vi "Create.vi"(8 "error in (no error)":errorcluster, 10 "Cylinder Types":T1, 11 "Actuator Cylinder Factory in":refnum<class "Actuator Cylinder Factory.lvclass">) -> (0 "error out":errorcluster, 2 "Actuator Cylinder":refnum<class "Actuator Cylinder.lvclass">, 3 "Actuator Cylinder Factory out":refnum<class "Actuator Cylinder Factory.lvclass">)   [LabVIEW 2015, in "Actuator Cylinder Factory.lvclass"]
uses:
  Actuator Cylinder Factory.lvclass
  Actuator Cylinder/Actuator Cylinder.lvclass
  Typedefs/Cylinder Types.ctl
  ILC DAC/ILC DAC Factory/ILC DAC Factory.lvclass
  ILC PSV Open Loop Actuator Cylinder/ILC PSV Open Loop Actuator Cylinder.lvclass
  ILC PSV Closed Loop Actuator Cylinder/ILC PSV Closed Loop Actuator Cylinder.lvclass
  ILC TV Open Loop Actuator Cylinder/ILC TV Open Loop Actuator Cylinder.lvclass
  ILC TV Closed Loop Actuator Cylinder/ILC TV Closed Loop Actuator Cylinder.lvclass
  ILC Closed Loop Actuator Cylinder/ILC Closed Loop Actuator Cylinder.lvclass
  ILC Actuator Cylinder/ILC Actuator Cylinder.lvclass/ILC Actuator Cylinder.ctl
  ILC Actuator Cylinder/ILC Actuator Cylinder.lvclass
  Boot Loader/Boot Loader.lvclass
  Typedefs/FAMT Typedefs.lvlib
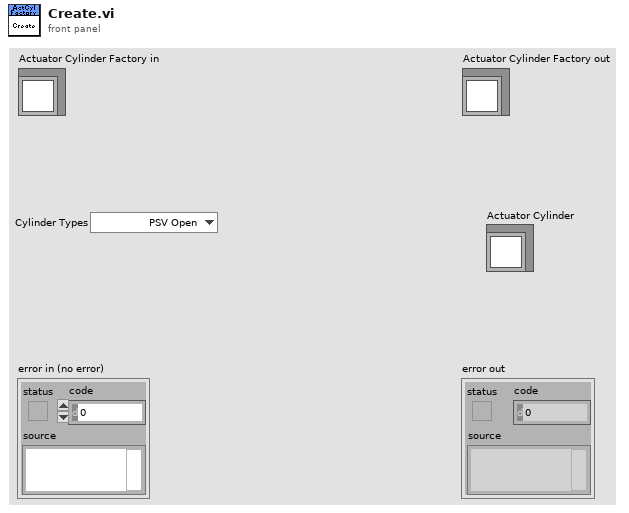
[diagram p1: front panel]
types:
  T1 = typedef "FAMT Typedefs.lvlib/Cylinder Types.ctl" = enum16{"PSV Open", "PSV Closed", "TV Open", "TV Closed", "Closed"}
  T2 = typedef "FAMT Typedefs.lvlib/Connection Settings.ctl" = cluster{"Pressure Servo Valve 1 DAC":u8, "Pressure Servo Valve 2 DAC":u8, "Flow Control Valve DAC":u8, "Load Cell ADC":u8, "FC1 ILC Port":refnum<visa-resource-name>, "FC2 ILC Port":refnum<visa-resource-name>, "Tovey A-B Port":refnum<visa-resource-name>, "Tovey C-D Port":refnum<visa-resource-name>, "Tovey E-F Port":refnum<visa-resource-name>, "FC1 ILC Protocol":T3, "FC2 ILC Protocol":T3, "Tovey A-B Protocol":T3, "Tovey C-D Protocol":T3, "Tovey E-F Protocol":T3, "Tovey A-B Address":u8, "Tovey C-D Address":u8, "Tovey E-F Address":u8}
  T3 = typedef "SerialProtocols.lvlib/SerialProtocol.ctl" = enum16{"RS232", "RS485", "SerialSimulator"}
  T4 = typedef "FAMT Typedefs.lvlib/Pressure Servo Valve Settings.ctl" = cluster{"Center Point":dbl[unit], "Area":dbl, "PA to PSI":dbl, "Off Value":dbl}
  T5 = typedef "FAMT Typedefs.lvlib/Turbo Valve Settings.ctl" = cluster{"ROT Bias":u8, "Minimum Voltage":dbl, "Maximum Voltage":dbl, "Off Value":dbl}
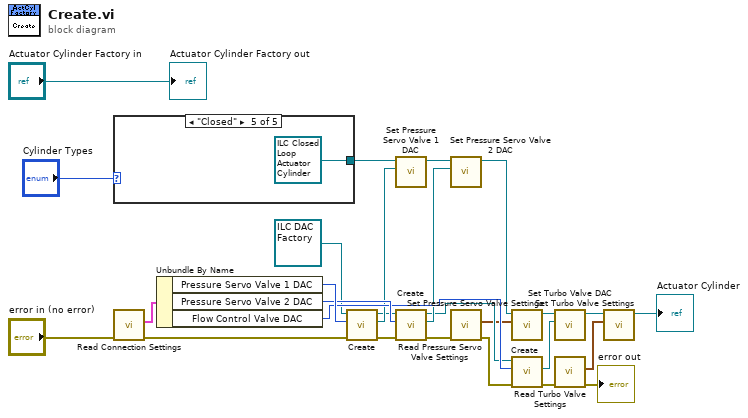
[diagram p0: block diagram]
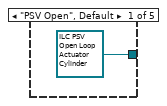
[diagram p2: hidden frame]
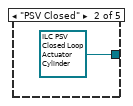
[diagram p3: hidden frame]
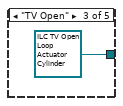
[diagram p4: hidden frame]
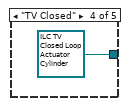
[diagram p5: hidden frame]
diagram:
  n1 = case shown="\"Closed\"" "Cylinder Types" {
    tunnel: [refnum<class "ILC PSV Open Loop Actuator Cylinder.lvclass"> refnum ("ILCPSVOpenLoopActuatorCylinder.lvclass") refnum<class "ILC PSV Closed Loop Actuator Cylinder.lvclass"> refnum ("ILCPSVClosedLoopActuatorCylinder.lvclass") refnum<class "ILC TV Open Loop Actuator Cylinder.lvclass"> refnum ("ILCTVOpenLoopActuatorCylinder.lvclass") refnum<class "ILC TV Closed Loop Actuator Cylinder.lvclass"> refnum ("ILCTVClosedLoopActuatorCylinder.lvclass") refnum<class "ILC Closed Loop Actuator Cylinder.lvclass"> refnum ("ILCClosedLoopActuatorCylinder.lvclass")] -> w25
    frame "PSV Open", Default {
    }
    frame "PSV Closed" {
    }
    frame "TV Open" {
    }
    frame "TV Closed" {
    }
    frame "Closed" {
    }
  }
  n2 = call "Read Connection Settings.vi"("error in (no error)"="error in (no error)") -> ("error out"=w8:errorcluster, "Connection Settings"=w7:T2)  [unwired: 8 in, 1 out]
  n3 = Unbundle By Name(w7) -> ("Pressure Servo Valve 1 DAC"=w19:u8, "Pressure Servo Valve 2 DAC"=w18:u8, "Flow Control Valve DAC"=w17:u8)
  n4 = call-dynamic "Create.vi"("error in (no error)"=w8, "Channel"=w19, "ILC DAC Factory in"=refnum<class "ILC DAC Factory.lvclass"> refnum ("ILCDACFactory.lvclass")) -> ("error out"=w10:errorcluster, "ILC DAC"=w14:refnum<class "ILC DAC.lvclass">, "ILC DAC Factory out"=w12:refnum<class "ILC DAC Factory.lvclass">)  [unwired: 6 in]
  n5 = call "Set Pressure Servo Valve 1 DAC.vi"("ILC DAC"=w14, "ILC Actuator Cylinder in"=w25) -> ("ILC Actuator Cylinder out"=w24:refnum<class "ILC Actuator Cylinder.lvclass">)  [unwired: 9 in]
  n6 = call-dynamic "Create.vi"("error in (no error)"=w10, "Channel"=w18, "ILC DAC Factory in"=w12) -> ("error out"=w6:errorcluster, "ILC DAC"=w15:refnum<class "ILC DAC.lvclass">, "ILC DAC Factory out"=w11:refnum<class "ILC DAC Factory.lvclass">)  [unwired: 6 in]
  n7 = call "Set Pressure Servo Valve 2 DAC.vi"("ILC DAC"=w15, "ILC Actuator Cylinder in"=w24) -> ("ILC Actuator Cylinder out"=w23:refnum<class "ILC Actuator Cylinder.lvclass">)  [unwired: 9 in]
  n8 = call "Read Pressure Servo Valve Settings.vi"("error in (no error)"=w6) -> ("error out"=w5:errorcluster, "Pressure Servo Valve Settings"=w4:T4)  [unwired: 8 in, 1 out]
  n9 = call "Set Pressure Servo Valve Settings.vi"("Pressure Servo Settings"=w4, "ILC Actuator Cylinder in"=w23) -> ("ILC Actuator Cylinder out"=w22:refnum<class "ILC Actuator Cylinder.lvclass">)  [unwired: 9 in]
  n10 = call-dynamic "Create.vi"("error in (no error)"=w5, "Channel"=w17, "ILC DAC Factory in"=w11) -> ("error out"=w3:errorcluster, "ILC DAC"=w16:refnum<class "ILC DAC.lvclass">)  [unwired: 6 in, 1 out]
  n11 = call "Set Turbo Valve DAC.vi"("IILCDAC"=w16, "ILC Actuator Cylinder in"=w22) -> ("ILC Actuator Cylinder out"=w21:refnum<class "ILC Actuator Cylinder.lvclass">)  [unwired: 9 in]
  n12 = call "Read Turbo Valve Settings.vi"("error in (no error)"=w3) -> ("error out"=→"error out":errorcluster, "Turbo Valve Settings"=w1:T5)  [unwired: 8 in, 1 out]
  n13 = call "Set Turbo Valve Settings.vi"("Turbo Valve Settings"=w1, "ILC Actuator Cylinder in"=w21) -> ("ILC Actuator Cylinder out"=→"Actuator Cylinder":refnum<class "ILC Actuator Cylinder.lvclass">)  [unwired: 9 in]
  "Actuator Cylinder Factory out" <- "Actuator Cylinder Factory in"
